vi "Initialize OAuth for LinkedIn.vi"(9 "Scopes":string[](array[string])=["r_liteprofile", "r_emailaddress "], 10 "Client Secret":string, 11 "Client ID":string) -> (3 "Oauth2.LinkedIn":refnum<class "Oauth2.LinkedIn.lvclass">)   [LabVIEW 2020, in "Oauth2.LinkedIn.lvclass"]
uses:
  Oauth2.LinkedIn.lvclass
  C:/Data/1_Projects/CIGH_Oauth2/source/Oauth2/Oauth2.lvclass
  Oauth2/Oauth2.lvclass
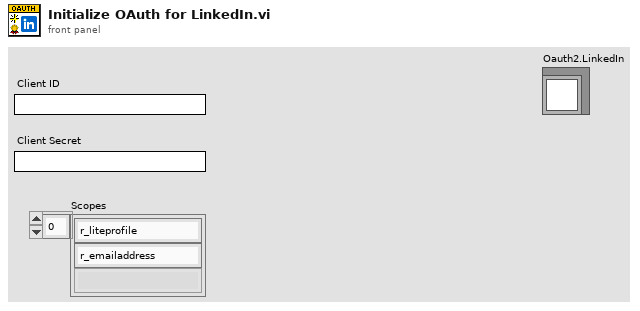
[diagram p1: front panel]
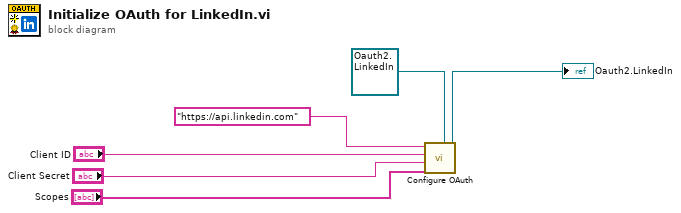
[diagram p0: block diagram]
diagram:
  n1 = call "Configure OAuth.vi"("Oauth2 in"=refnum<class "Oauth2.LinkedIn.lvclass"> refnum ("Oauth2.LinkedIn.lvclass"), "scopes"="Scopes", "Client Secret"="Client Secret", "Client ID"="Client ID", "Authorization Server URI"="https://api.linkedin.com") -> ("Oauth2"=→"Oauth2.LinkedIn":refnum<class "Oauth2.LinkedIn.lvclass">)  [unwired: 5 in, 1 out]
